vi "HighScore.vi"(8 "error in (no error)":errorcluster, 11 "tdms file":refnum<k34>) -> (0 "error out":errorcluster, 2 "Array":string[][](array[string]), 3 "tdms file out":refnum<k34>)   [LabVIEW 2022 SP3]
uses:
  <vilib>/Array/Sort 2D Array - Pop Stack.vi
  <vilib>/Array/Sort 2D Array - Push Stack.vi
  f4964591-22ec-4ef2-89ea-eaaee1989f18.vi
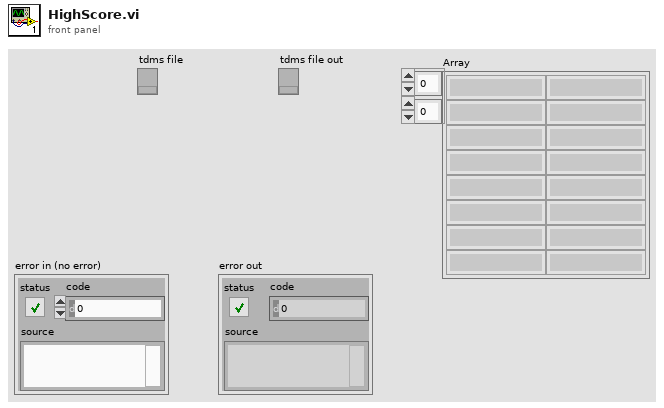
[diagram p1: front panel]
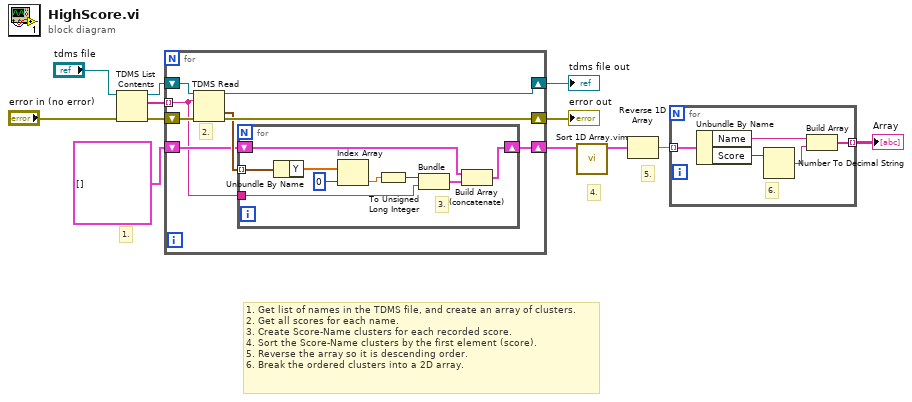
[diagram p0: block diagram]
diagram:
  # "5."
  # "4."
  # "1. Get list of names in the TDMS file, and create an array of clusters.\n2. Get all scores for each name.\n3. Create Score-Name clusters for each recorded score.\n4. Sort the Score-Name clusters by the first element (score).\n5. Reverse the array so it is descending order.\n6. Break the ordered clusters into a 2D array."
  # "1."
  n1 = TDMS List Contents(4:"error in (no error)", 7:"tdms file") -> (0:w10:errorcluster, 2:w12:string[], 3:w11:refnum<k34>)  [unwired: 1 in, 1 out]
  n2 = for {
    shift-right: [w18] -> w1
    shift-left: w11 -> [w20]
    shift-right: [w17] -> w2
    shift-left: w10 -> [w19]
    tunnel: w12 -> [w14] mode=indexing
    shift-right: [w13] -> w8
    shift-left: cluster{"Score":u32, "Name":string}[] [] -> [w15]
    # "2."
    n3 = TDMS Read(0:w20, 5:w14, 11:w19) -> (4:w18:refnum<k34>, 10:w16:waveform(dbl)[], 15:w17:errorcluster)  [unwired: 5 in, 3 out]
    n4 = for {
      tunnel: w16 -> [w29] mode=indexing
      shift-right: [w21] -> w13
      shift-left: w15 -> [w25]
      tunnel: w14 -> [w23]
      # "3."
      n5 = Unbundle By Name(w29) -> ("Y"=w28:dbl[])
      n6 = Index Array(array=w28, index=0) -> (element=w26:dbl)
      n7 = To Unsigned Long Integer(number=w26) -> (unsigned 32bit integer=w24:u32)
      n8 = Bundle(w24, w23) -> (w22:cluster{u32, string})  [unwired: 1 in]
      n9 = Build Array (concatenate)(w25, w22) -> (w21:cluster{"Score":u32, "Name":string}[])
    }
  }
  "error out" <- w2
  "tdms file out" <- w1
  n10 = call "Sort 1D Array.vim"("unsorted array"=w8) -> ("sorted array"=w7:cluster{"Score":u32, "Name":string}[])  [unwired: 10 in]
  n11 = Reverse 1D Array(array=w7) -> (reversed array=w6:cluster{"Score":u32, "Name":string}[])
  n12 = for {
    tunnel: w6 -> [w34] mode=indexing
    tunnel: [w30] -> w5 mode=indexing
    # "6."
    n13 = Unbundle By Name(w34) -> ("Name"=w32:string, "Score"=w33:u32)
    n14 = Number To Decimal String(number=w33) -> (decimal integer string=w31:string)  [unwired: 1 in]
    n15 = Build Array(w32, w31) -> (w30:string[])
  }
  "Array" <- w5
